vi "CalcCRC.vi"(8 "error in (no error)":errorcluster, 10 "TextIn":string, 11 "reference in":refnum<class "VdMultiMeter.lvclass">) -> (0 "error out":errorcluster, 2 "CrcOut":string, 3 "reference out":refnum<class "VdMultiMeter.lvclass">)   [LabVIEW 2020, in "MulitMeters.lvlib" / "VdMultiMeter.lvclass"]
uses:
  VdMultiMeter.lvclass
  VdMultiMeter.lvclass/VdMultiMeter.ctl
  ChecksumCalculation_interface/ChecksumCalculation.lvclass
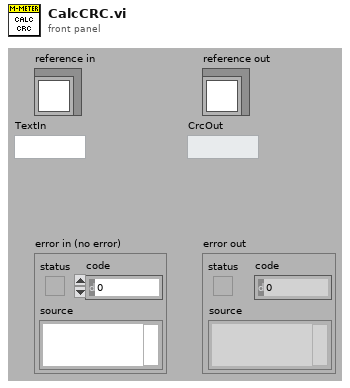
[diagram p1: front panel]
types:
  T1 = typedef "MulitMeters.lvlib/VdMultiMeter.lvclass/ObjectAttributes.ctl" = cluster{"ChecksumCalculationType":refnum<class "ChecksumCalculation.lvclass">}
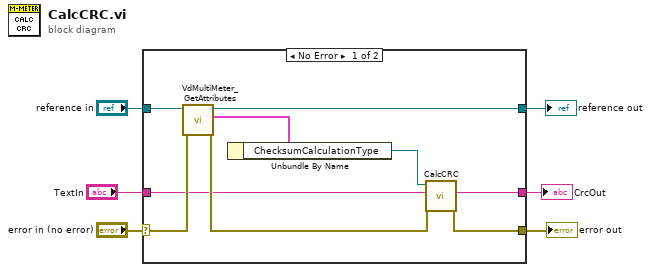
[diagram p0: block diagram]
diagram:
  n1 = case shown="No Error" "error in (no error)" {
    selector: "error in (no error)" -> [w15 w17]
    tunnel: [w10 w17] -> w5
    tunnel: [w12 w16] -> w3
    tunnel: "reference in" -> [w13 w16]
    tunnel: "TextIn" -> [w9 _]
    tunnel: [w8 _] -> w1
    frame No Error {
      n2 = call "VdMultiMeter_GetAttributes.vi"("error in (no error)"=w15, "reference in"=w13) -> ("error out"=w11:errorcluster, "Data"=w14:T1, "reference out"=w12:refnum<class "VdMultiMeter.lvclass">)  [unwired: 6 in, 1 out]
      n3 = Unbundle By Name(w14) -> ("ChecksumCalculationType"=w7:refnum<class "ChecksumCalculation.lvclass">)
      n4 = call-dynamic "CalcCRC.vi"("error in (no error)"=w11, "TextIn"=w9, "object in"=w7) -> ("error out"=w10:errorcluster, "CrcOut"=w8:string)  [unwired: 6 in, 1 out]
    }
    frame Error {
    }
  }
  "error out" <- w5
  "reference out" <- w3
  "CrcOut" <- w1
